vi "Drive Immediate.vi"(7 "Description":string, 8 "Command Info In":T2, 11 "Robot Velocities":T1) -> (0 "Command Info Out":T2)   [LabVIEW 2020]
doc: "Often used for joystick control, this VI checks to see that the joystick axes are outside the deadband and updates the motors appropriately."
uses:
  Implementation/Drive Operations.ctl
  Implementation/Drive Setpoints.ctl
  swerve/Type Definitions/Data/Robot Velocities.ctl
  <vilib>/Rock Robotics/WPI/Framework/Completion Status.ctl
  <vilib>/Rock Robotics/WPI/Framework/Completion Notifier.ctl
  <vilib>/Rock Robotics/WPI/Framework/Command Status Info.ctl
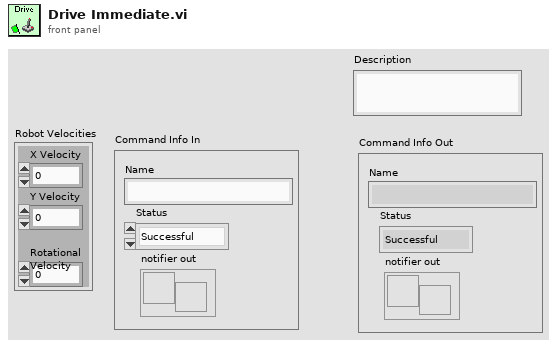
[diagram p1: front panel]
types:
  T1 = typedef "Robot Velocities.ctl" = cluster{"X Velocity":dbl, "Y Velocity":dbl, "Rotational \nVelocity":dbl}
  T2 = typedef "Command Status Info.ctl" = cluster{"Name":string, "Status":T3, "notifier out":T4}
  T3 = typedef "Completion Status.ctl" = enum16{"Successful", "Aborted", "Incomplete"}
  T4 = typedef "Completion Notifier.ctl" = refnum<notifier>
  T5 = typedef "Drive Setpoints.ctl" = cluster{"Operation":T6, "Robot Velocities":T1, "Auto Data":cluster{"Auto Velocities":T1[], "Auto Positions":cluster{"x":dbl, "y":dbl, "th":dbl}[], "Auto Commands":cluster{dbl, "Command out":cluster{"Name":string, "vi reference":refnum<vi>, i32[], variant[]}}[], "Zero Velocity?":bool[]}}
  T6 = typedef "Drive Operations.ctl" = enum16{"Reserve", "Read Current", "Immediate", "Calibrate", "Auto", "Brake"}
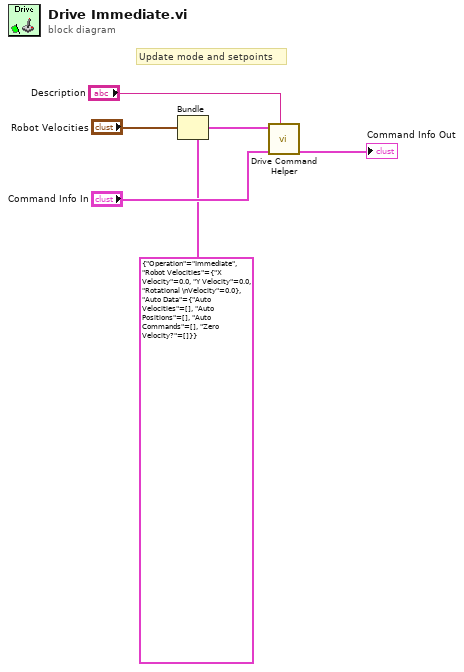
[diagram p0: block diagram]
diagram:
  # "Update mode and setpoints"
  n1 = Bundle(cluster=T5 {"Operation"=enum."Immediate", "Robot Velocities"={"X Velocity"=0.0, "Y Velocity"=0.0, "Rotational \nVelocity"=0.0}, "Auto Data"={"Auto Velocities"=[], "Auto Positions"=[], "Auto Commands"=[], "Zero Velocity?"=[]}} ("SubSystem Data"), "Robot Velocities"="Robot Velocities") -> (w2:T5)  [unwired: 2 in]
  n2 = call "Drive Command Helper.vi"("Description"="Description", "Command Info In"="Command Info In", "SubSystem Data"=w2) -> ("Command Info Out"=→"Command Info Out":T2)  [unwired: 6 in, 2 out]
